vi "Score and Rank Target Objects.vi"(8 "Annotate":bool, 9 "Score Limit":dbl=70.0, 10 "Particles":T4(array[cluster]), 11 "Image in":T3) -> (0 "Target Info":T2(array[cluster]), 3 "Annotated Image":T3)   [LabVIEW 2013]
doc: "Use the location, size, and other factors to score and rank the objects. Optionally show annotations over the objects."
uses:
  <vilib>/vision/Image Controls.llb/IMAQ Image.ctl
  TargetType.ctl
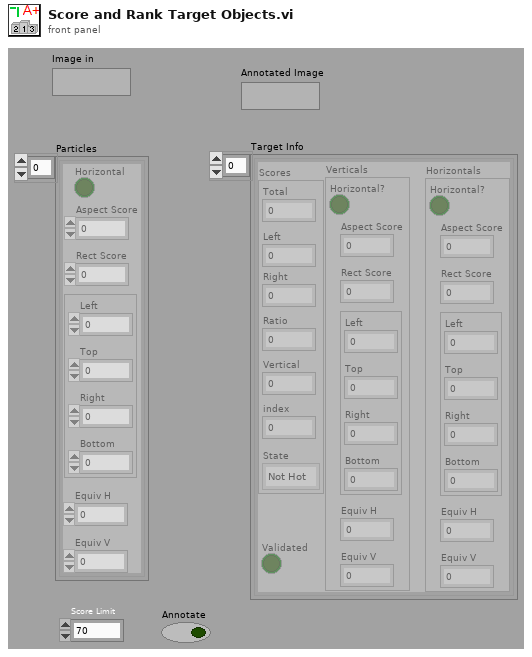
[diagram p1: front panel]
types:
  T1 = typedef "TargetType.ctl" = enum16{"Not Hot", "Hot"}
  T2 = cluster{"Scores":cluster{"Total":dbl, "Left":dbl, "Right":dbl, "Ratio":dbl, "Vertical":dbl, "index":i32, "State":T1}, "Verticals":cluster{"Horizontal?":bool, "Aspect Score":dbl, "Rect Score":dbl, cluster{"Left":dbl, "Top":dbl, "Right":dbl, "Bottom":dbl}, "Equiv H":dbl, "Equiv V":dbl}, "Horizontals":cluster{"Horizontal?":bool, "Aspect Score":dbl, "Rect Score":dbl, cluster{"Left":dbl, "Top":dbl, "Right":dbl, "Bottom":dbl}, "Equiv H":dbl, "Equiv V":dbl}, "Validated":bool}[]
  T3 = typedef "IMAQ Image.ctl" = refnum<image>
  T4 = cluster{"Horizontal":bool, "Aspect Score":dbl, "Rect Score":dbl, cluster{"Left":dbl, "Top":dbl, "Right":dbl, "Bottom":dbl}, "Equiv H":dbl, "Equiv V":dbl}[]
  T5 = cluster{cluster{dbl, dbl, dbl, dbl, dbl, i32, T1}, cluster{"Horizontal":bool, "Aspect Score":dbl, "Rect Score":dbl, cluster{"Left":dbl, "Top":dbl, "Right":dbl, "Bottom":dbl}, "Equiv H":dbl, "Equiv V":dbl}, cluster{"Horizontal":bool, "Aspect Score":dbl, "Rect Score":dbl, cluster{"Left":dbl, "Top":dbl, "Right":dbl, "Bottom":dbl}, "Equiv H":dbl, "Equiv V":dbl}, bool}[]
  T6 = cluster{"Score":dbl, cluster{"Horizontal":bool, "Aspect Score":dbl, "Rect Score":dbl, cluster{"Left":dbl, "Top":dbl, "Right":dbl, "Bottom":dbl}, "Equiv H":dbl, "Equiv V":dbl}}[]
  T7 = cluster{"Horizontal":bool, "Aspect Score":dbl, "Rect Score":dbl, cluster{"Left":dbl, "Top":dbl, "Right":dbl, "Bottom":dbl}, "Equiv H":dbl, "Equiv V":dbl}
  T8 = cluster{cluster{dbl, dbl, dbl, dbl, dbl, i32, T1}, cluster{"Horizontal":bool, "Aspect Score":dbl, "Rect Score":dbl, cluster{"Left":dbl, "Top":dbl, "Right":dbl, "Bottom":dbl}, "Equiv H":dbl, "Equiv V":dbl}, cluster{"Horizontal":bool, "Aspect Score":dbl, "Rect Score":dbl, cluster{"Left":dbl, "Top":dbl, "Right":dbl, "Bottom":dbl}, "Equiv H":dbl, "Equiv V":dbl}, bool}
  T9 = cluster{"Score":dbl, cluster{"Horizontal":bool, "Aspect Score":dbl, "Rect Score":dbl, cluster{"Left":dbl, "Top":dbl, "Right":dbl, "Bottom":dbl}, "Equiv H":dbl, "Equiv V":dbl}}
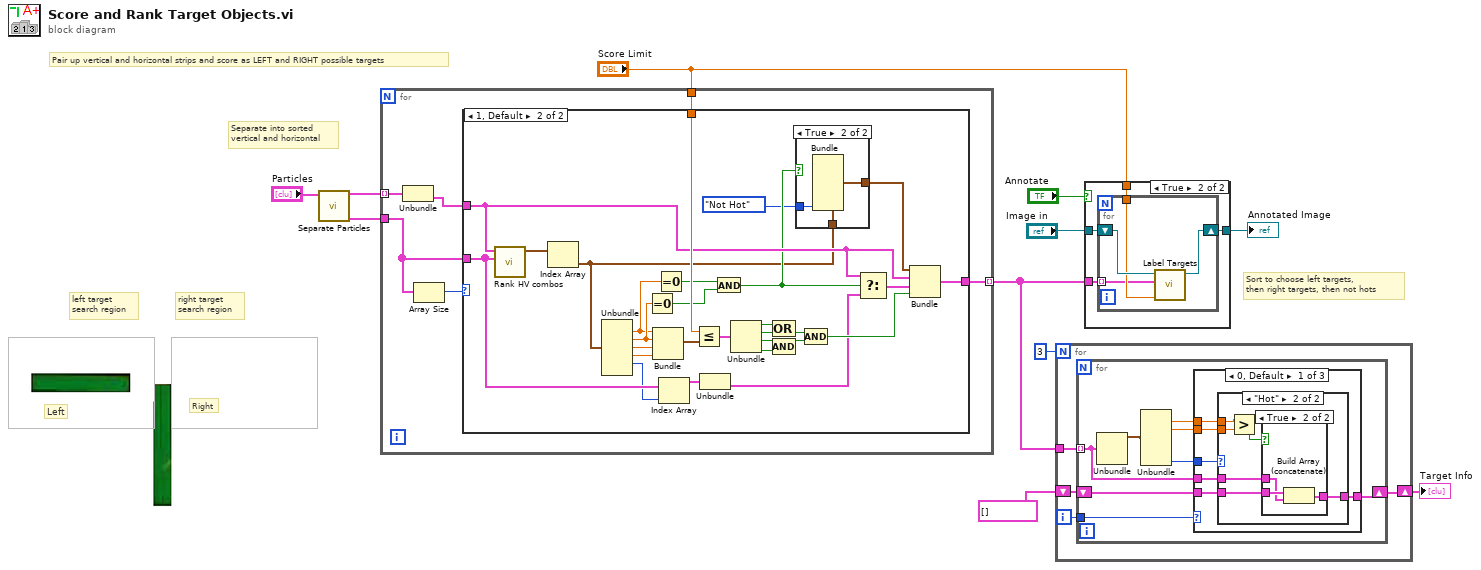
[diagram p0: block diagram]
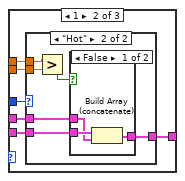
[diagram p5: hidden frame]
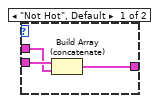
[diagram p9: hidden frame]
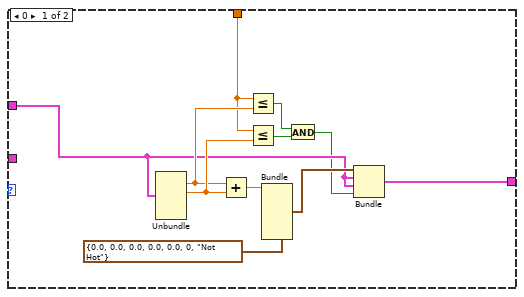
[diagram p10: hidden frame]
diagram:
  # "Sort to choose left targets,\nthen right targets, then not hots"
  # "Right"
  # "Left"
  # "right target\nsearch region"
  # "left target\nsearch region"
  # "Separate into sorted\nvertical and horizontal"
  # "Pair up vertical and horizontal strips and score as LEFT and RIGHT possible targets"
  n1 = call "Separate Particles.vi"("Objects"="Particles") -> ("H Scores"=w7:T6, "V Scores"=w8:T6)  [unwired: 9 in]
  n2 = for {
    tunnel: w8 -> [w17] mode=indexing
    tunnel: w7 -> [w15]
    tunnel: [w13] -> w5 mode=indexing
    tunnel: "Score Limit" -> [w12]
    n3 = Unbundle(w17) -> (w16:T7)  [unwired: 1 out]
    n4 = Array Size(array=w15) -> (size(s)=w14:i32)
    n5 = case shown="1, Default" w14 {
      tunnel: w15 -> [_ w43]
      tunnel: w16 -> [w22 w33]
      tunnel: [w20 w41] -> w13
      tunnel: w12 -> [w19 w40]
      frame 0 {
        n6 = Unbundle(w22) -> ("Aspect Score"=w25:dbl, "Rect Score"=w26:dbl)  [unwired: 4 out]
        n7 = Add(x=w25, y=w26) -> (x+y=w24:dbl)
        n8 = Less Or Equal?(x=w19, y=w25) -> (x <= y?=w27:bool)
        n9 = Less Or Equal?(x=w19, y=w26) -> (x <= y?=w28:bool)
        n10 = Bundle(cluster=cluster{dbl, dbl, dbl, dbl, dbl, i32, T1} {0.0, 0.0, 0.0, 0.0, 0.0, 0, enum."Not Hot"}, w24) -> (w23:cluster{dbl, dbl, dbl, dbl, dbl, i32, T1})  [unwired: 6 in]
        n11 = And(x=w27, y=w28) -> (x .and. y?=w21:bool)
        n12 = Bundle(w23, w22, w22, w21) -> (w20:T8)  [unwired: 1 in]
      }
      frame 1, Default {
        n13 = call "Rank HV combos.vi"("H Scores"=w43, "Vertical"=w33) -> ("Target Scores"=w56:cluster{dbl, dbl, dbl, dbl, dbl, i32, T1}[])  [unwired: 9 in]
        n14 = Index Array(array=w56) -> (element=w29:cluster{dbl, dbl, dbl, dbl, dbl, i32, T1})  [unwired: 1 in]
        n15 = Unbundle(w29) -> (w38:dbl, w39:dbl, w52:dbl, w53:dbl, w42:i32)  [unwired: 2 out]
        n16 = Equal To 0?(x=w39) -> (x = 0?=w36:bool)
        n17 = Bundle(w38, w39, w52, w53) -> (w44:cluster{dbl, dbl, dbl, dbl})  [unwired: 1 in]
        n18 = Equal To 0?(x=w38) -> (x = 0?=w37:bool)
        n19 = Index Array(array=w43, index=w42) -> (element=w54:T9)
        n20 = Less Or Equal?(x=w40, y=w44) -> (x <= y?=w51:cluster{bool, bool, bool, bool})
        n21 = Unbundle(w54) -> (w34:T7)  [unwired: 1 out]
        n22 = And(x=w37, y=w36) -> (x .and. y?=w32:bool)
        n23 = Unbundle(w51) -> (w50:bool, w49:bool, w48:bool, w47:bool)
        n24 = Compound Arithmetic op=OR(w50, w49) -> (w45:bool)
        n25 = Compound Arithmetic op=AND(w48, w47) -> (w46:bool)
        n26 = case shown="True" w32 {
          tunnel: w29 -> [w57 w60]
          tunnel: TargetType."Not Hot" -> [_ w59]
          tunnel: [w57 w58] -> w30
          frame False {
          }
          frame True {
            n27 = Bundle(cluster=w60, w59) -> (w58:cluster{dbl, dbl, dbl, dbl, dbl, i32, T1})  [unwired: 6 in]
          }
        }
        n28 = Compound Arithmetic op=AND(w45, w46) -> (w55:bool)
        n29 = Select(t=w33, s=w32, f=w34) -> (s? t:f=w35:T7)
        n30 = Bundle(w30, w33, w35, w55) -> (w41:T8)  [unwired: 1 in]
      }
    }
  }
  n31 = for {
    N: 3 -> [_]
    tunnel: w5 -> [w64]
    shift-right: [w61] -> w3
    shift-left: T5 [] -> [w62]
    i -> [w63]
    n32 = for {
      tunnel: w64 -> [w68] mode=indexing
      tunnel: w63 -> [w67]
      shift-right: [w65] -> w61
      shift-left: w62 -> [w66]
      n33 = Unbundle(w68) -> (w72:cluster{dbl, dbl, dbl, dbl, dbl, i32, T1})  [unwired: 3 out]
      n34 = Unbundle(w72) -> (w71:dbl, w70:dbl, w69:T1)  [unwired: 4 out]
      n35 = case shown="0, Default" w67 {
        tunnel: w71 -> [w78 w92 w112]
        tunnel: w70 -> [w77 w91 w111]
        tunnel: w69 -> [w74 w90 w110]
        tunnel: w68 -> [w73 w95 w109]
        tunnel: w66 -> [w76 w94 w108]
        tunnel: [w75 w93 w107] -> w65
        frame 0, Default {
          n36 = case shown="\"Hot\"" w74 {
            tunnel: w76 -> [w79 w83]
            tunnel: [w79 w81] -> w75
            tunnel: w78 -> [_ w85]
            tunnel: w77 -> [_ w84]
            tunnel: w73 -> [_ w80]
            frame "Not Hot", Default {
            }
            frame "Hot" {
              n37 = Greater?(x=w85, y=w84) -> (0:w82:bool)
              n38 = case shown="True" w82 {
                tunnel: w83 -> [w86 w89]
                tunnel: [w86 w88] -> w81
                tunnel: w80 -> [_ w87]
                frame False {
                }
                frame True {
                  n39 = Build Array (concatenate)(w89, w87) -> (w88:T5)
                }
              }
            }
          }
        }
        frame 1 {
          n40 = case shown="\"Hot\"" w90 {
            tunnel: w94 -> [w96 w100]
            tunnel: [w96 w98] -> w93
            tunnel: w92 -> [_ w102]
            tunnel: w91 -> [_ w101]
            tunnel: w95 -> [_ w97]
            frame "Not Hot", Default {
            }
            frame "Hot" {
              n41 = Greater?(x=w102, y=w101) -> (0:w99:bool)
              n42 = case shown="False" w99 {
                tunnel: w100 -> [w105 w106]
                tunnel: [w104 w106] -> w98
                tunnel: w97 -> [w103 _]
                frame False {
                  n43 = Build Array (concatenate)(w105, w103) -> (w104:T5)
                }
                frame True {
                }
              }
            }
          }
        }
        frame 2 {
          n44 = case shown="\"Hot\"" w110 {
            tunnel: w112 -> [_ _]
            tunnel: w111 -> [_ _]
            tunnel: w109 -> [w114 _]
            tunnel: w108 -> [w115 w116]
            tunnel: [w113 w116] -> w107
            frame "Not Hot", Default {
              n45 = Build Array (concatenate)(w115, w114) -> (w113:T5)
            }
            frame "Hot" {
            }
          }
        }
      }
    }
  }
  "Target Info" <- w3
  n46 = case shown="True" "Annotate" {
    tunnel: "Image in" -> [w117 w121]
    tunnel: [w117 w120] -> w10
    tunnel: "Score Limit" -> [_ w119]
    tunnel: w5 -> [_ w118]
    frame False {
    }
    frame True {
      n47 = for {
        shift-right: [w122] -> w120
        shift-left: w121 -> [w125]
        tunnel: w118 -> [w123] mode=indexing
        tunnel: w119 -> [w124]
        n48 = call "Label Targets.vi"("Score Limit"=w124, "Target Info"=w123, "Image in"=w125) -> ("Image out"=w122:T3)  [unwired: 8 in]
      }
    }
  }
  "Annotated Image" <- w10
